vi "SetProcessRunId.vi"(8 "error in":errorcluster, 10 "ProcessRunId":string, 11 "ProcessRun in":refnum<class "ProcessRun.lvclass">) -> (0 "error out":errorcluster, 3 "ProcessRun out":refnum<class "ProcessRun.lvclass">)   [LabVIEW 2021, in "ProligentXMLGenerator.lvlib" / "ProcessRun.lvclass"]
doc: "Defines an ID for this process run. This ID should be reused when providing results for a process run spanned over multiple files. If no ProcessRunId is provided, all the results of this process run must be provided in the context of a single ProcessRun."
uses:
  ProcessRun.lvclass
  ProcessRun.lvclass/ProcessRun.ctl
  Base/Attribute/Attribute.lvclass
  Base/Guid/Guid.lvclass
  C:/Projects/proligent-xml-generator-labview/src/ProligentXMLGenerator/Base/NonEmptyString/NonEmptyString.lvclass
  C:/Projects/proligent-xml-generator-labview/src/ProligentXMLGenerator/Base/String/String.lvclass
  C:/Projects/proligent-xml-generator-labview/src/ProligentXMLGenerator/Base/Attribute/Attribute.lvclass
  C:/Projects/proligent-xml-generator-labview/src/ProligentXMLGenerator/Base/Guid/Guid.lvclass
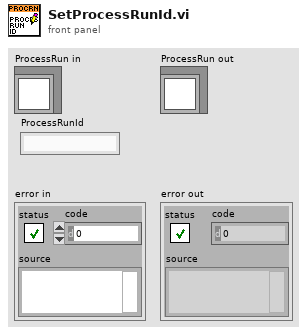
[diagram p1: front panel]
types:
  T1 = typedef "ProligentXMLGenerator.lvlib/ProcessRun.lvclass/Data.ctl" = cluster{"Name":string, "OperationRuns":refnum<class "OperationRun.lvclass">[], "OperationCycles":refnum<class "OperationCycle.lvclass">[], "FailureReferences":refnum<class "FailureReference.lvclass">[], "CustomData":refnum<class "CustomData.lvclass">, "ProcessRunId":refnum<class "Guid.lvclass">, "ProcessFullName":refnum<class "ProcessFullName.lvclass">, "ProcessVersion":refnum<class "NonEmptyString_64.lvclass">, "ProductUnitIdentifier":refnum<class "NonEmptyString_50.lvclass">, "ProductFullName":refnum<class "FullName.lvclass">, "ProcessRunStatus":refnum<class "ExecutionStatus.lvclass">, "ProcessRunStartTime":refnum<class "DateTime.lvclass">, "ProcessRunEndTime":refnum<class "DateTime.lvclass">, "ProcessMode":refnum<class "NonEmptyString_64.lvclass">, "TimeZoneInfoId":string}
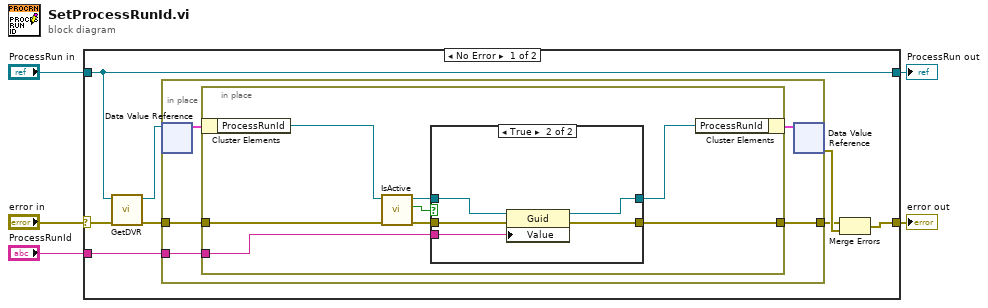
[diagram p0: block diagram]
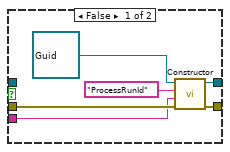
[diagram p2: hidden frame]
diagram:
  n1 = case shown="No Error" "error in" {
    selector: "error in" -> [w11 w38]
    tunnel: "ProcessRun in" -> [w6 w39]
    tunnel: [w8 w38] -> w3
    tunnel: "ProcessRunId" -> [w7 _]
    tunnel: [w6 w39] -> w1
    frame No Error {
      n2 = call "GetDVR.vi"("error in"=w11, "ProcessRun"=w6) -> ("error out"=w10:errorcluster, "DVRReference"=w12:refnum<data-value>)  [unwired: 8 in]
      n3 = in-place "In Place Element Structure" {
        in-place-border: w10 -> [w18]
        in-place-border: [w17] -> w9
        in-place-border: w7 -> [w16]
        n4 = in-place-dvr #1(w12) -> (w15:T1)  [unwired: 1 out]
        n5 = in-place "In Place Element Structure" {
          in-place-border: w18 -> [w23]
          in-place-border: [w26] -> w17
          in-place-border: w16 -> [w25]
          n6 = in-place-cluster #2(w15) -> ("ProcessRunId"=w21:refnum<class "Guid.lvclass">)
          n7 = call "IsActive.vi"("error in"=w23, "Attribute in"=w21) -> ("error out"=w24:errorcluster, "IsActive"=w22:bool, "Attribute in"=w20:refnum<class "Guid.lvclass">)  [unwired: 7 in]
          n8 = case shown="True" w22 {
            tunnel: w24 -> [w28 w37]
            tunnel: [w29 w36] -> w26
            tunnel: w25 -> [w27 w35]
            tunnel: [w31 w33] -> w19
            tunnel: w20 -> [_ w34]
            frame False {
              n9 = call-dynamic "Constructor.vi"("error in"=w28, "Value"=w27, "Name"="ProcessRunId", "String in"=refnum<class "Guid.lvclass"> refnum ("ProligentResultProcessor:Guid.lvclass")) -> ("error out"=w29:errorcluster, "String out"=w31:refnum<class "Guid.lvclass">)  [unwired: 6 in]
            }
            frame True {
              n10 = property on="Property Node" class="Guid"(reference=w34, error in=w37, "Value"=w35) -> (reference out=w33:refnum<class "Guid.lvclass">, error out=w36:errorcluster)
            }
          }
          n11 = in-place-cluster #2("ProcessRunId"=w19) -> (w14:T1)
        }
        n12 = in-place-dvr #1(w14) -> (w13:errorcluster)  [unwired: 1 out]
      }
      n13 = Merge Errors(w9, w13) -> (w8:errorcluster)
    }
    frame Error {
    }
  }
  "error out" <- w3
  "ProcessRun out" <- w1
